vi "libssh2_channel_handle_extended_data2.vi"(8 "error in (no error)":errorcluster, 10 "mode (normal)":i32(ring) items=["normal", "ignore", "merge"], 11 "channel":T1) -> (0 "error out":errorcluster)   [LabVIEW 2013, in "libssh2.lvlib"]
doc: "Set how extended data is handled on a channel."
uses:
  libssh2.lvlib
  Channel Refnum.ctl
  Acquire Session.vi
  Release Session.vi
  Not A Channel.vi
  <vilib>/Utility/error.llb/Error Cluster From Error Code.vi
  Global Settings.vi
  Read Channel Refnum.vi
  Read Session Refnum.vi
  <vilib>/Utility/semaphor.llb/Acquire Semaphore.vi
  <vilib>/Utility/semaphor.llb/Release Semaphore.vi
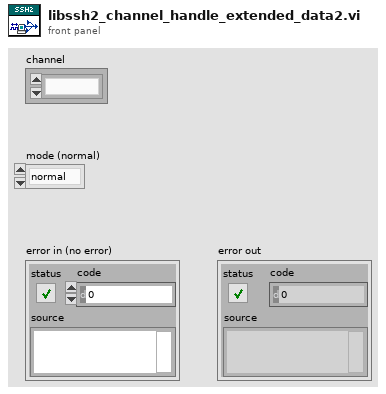
[diagram p1: front panel]
types:
  T1 = typedef "libssh2.lvlib/Channel Refnum.ctl" = refnum<k1>
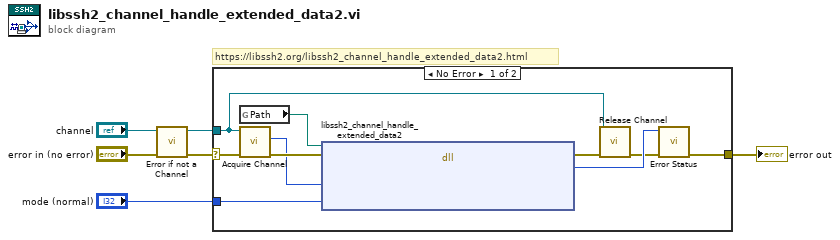
[diagram p0: block diagram]
diagram:
  # "https://libssh2.org/libssh2_channel_handle_extended_data2.html"
  n1 = call "Error if not a Channel.vi"("error in (no error)"="error in (no error)", "channel"="channel") -> ("error out"=w3:errorcluster, "channel out"=w1:T1)  [unwired: 8 in]
  n2 = case shown="No Error" w3 {
    selector: w3 -> [w15 w17]
    tunnel: [w10 w17] -> w6
    tunnel: "mode (normal)" -> [w11 _]
    tunnel: w1 -> [w7 _]
    frame No Error {
      n3 = global read "Global Settings.vi" "Path"() -> (w12:path)
      n4 = call "Acquire Channel.vi"("error in (no error)"=w15, "channel"=w7) -> ("error out"=w14:errorcluster, "LIBSSH2_CHANNEL*"=w13:u64)  [unwired: 8 in]
      n5 = dll-call lib="?" fn="libssh2_channel_handle_extended_data2"(path in=w12, error in=w14, "channel"=w13, "ignore_mode"=w11) -> (error out=w16:errorcluster, "return value"=w9:i32)  [unwired: 3 in, 1 out]
      n6 = call "Release Channel.vi"("error in (no error)"=w16, "channel"=w7) -> ("error out"=w8:errorcluster)  [unwired: 9 in]
      n7 = call "Error Status.vi"("error in (no error)"=w8, "return value"=w9) -> ("error out"=w10:errorcluster)  [unwired: 8 in, 1 out]
    }
    frame Error {
    }
  }
  "error out" <- w6
